vi "20220106_DO_Validation.vi"() -> ()   [LabVIEW 2021]
uses:
  <vilib>/Utility/file.llb/Read Delimited Spreadsheet (I64).vi
panel:
  out "Waveform Graph":waveform(i16)[](graph)
  out "Boolean array":bool[][](array[boolean])
  out "Waveform Chart":waveform(i64)(graph)
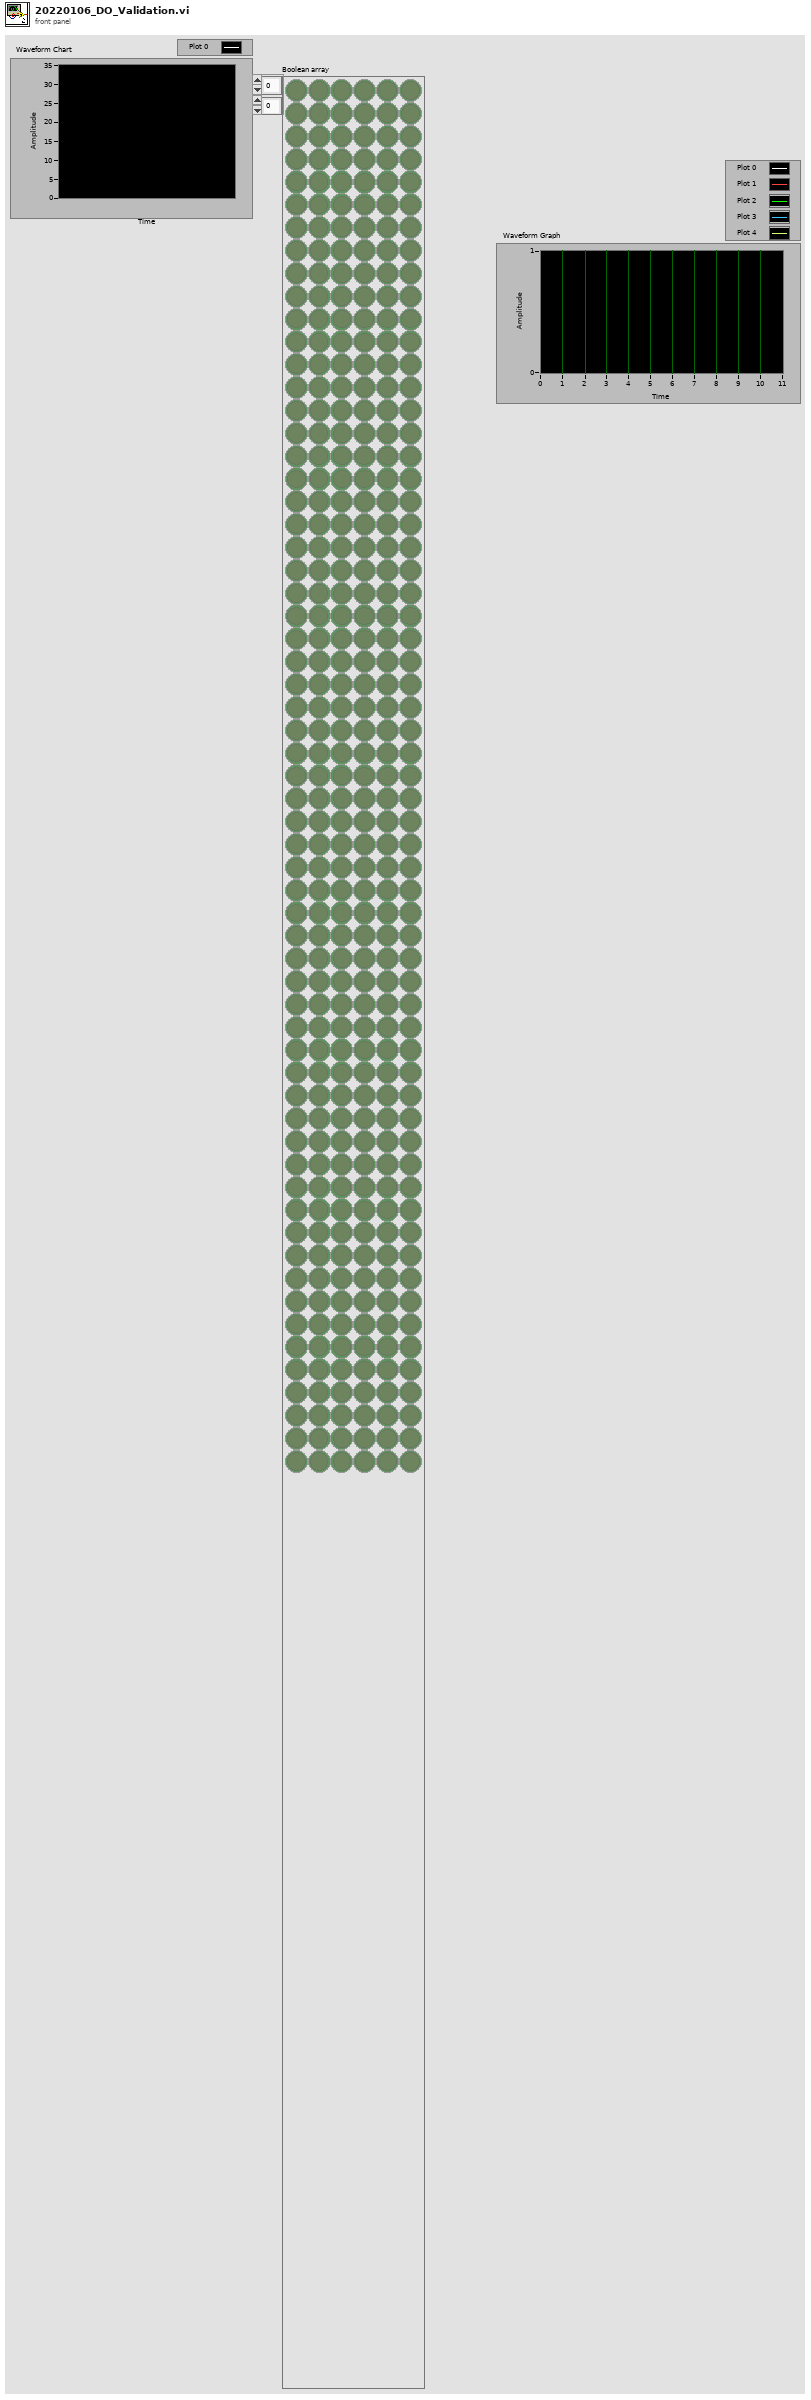
[diagram p1: front panel]
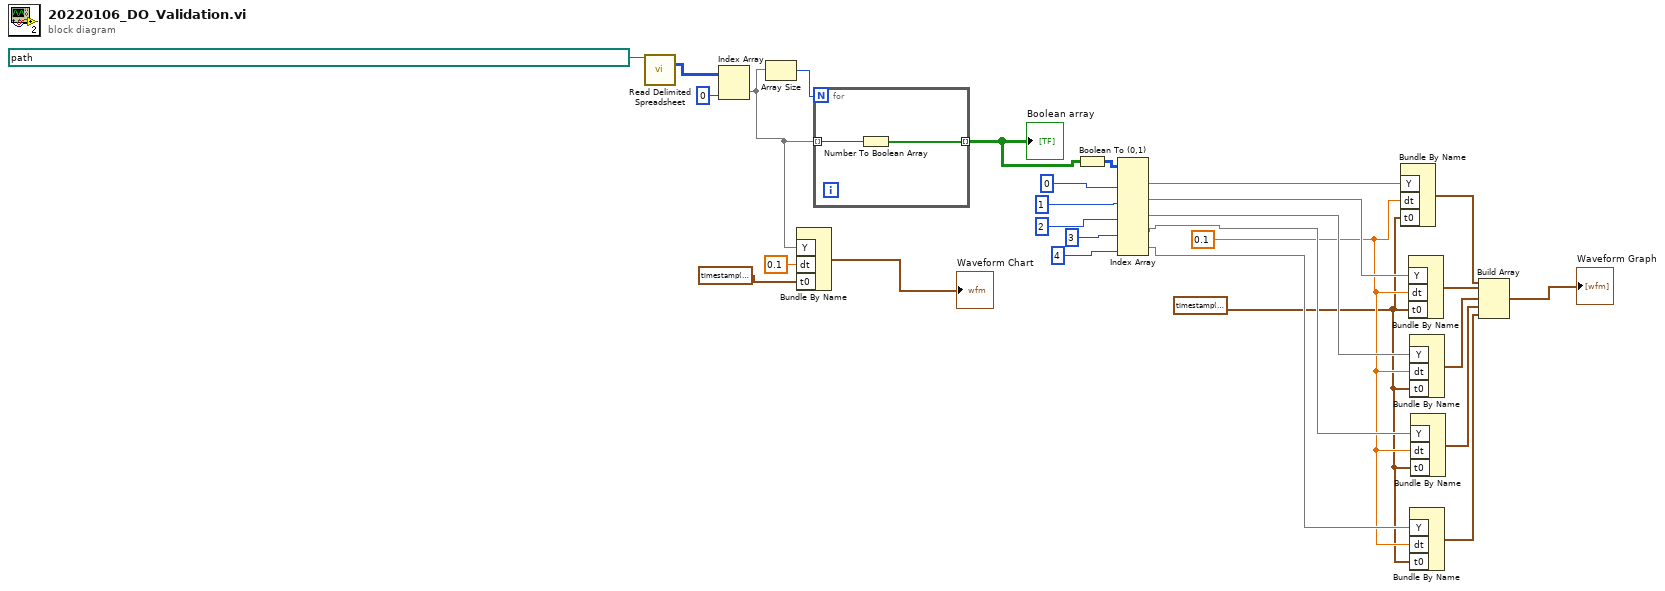
[diagram p0: block diagram]
diagram:
  w4 = timestamp(0 s since 1904-01-01) ("t0")
  w5 = 0.1 ("dt")
  n1 = call-poly <vilib>:"Read Delimited Spreadsheet.vi"("file path (dialog if empty)"=path "C:/Users/joe.kao/OneDrive - eCloudvalley Digital Technology/桌面/nPM1100_WaveformTable_Digital_LV.txt") -> ("all rows"=w27:i64[][])  [unwired: 9 in, 5 out]
  n2 = Index Array(array=w27, index (col)=0 ("disabled index (col)")) -> (element=w21:i64[])  [unwired: 1 in]
  n3 = Array Size(array=w21) -> (size(s)=w22:i32)
  n4 = Bundle By Name("Y"=w21, "dt"=0.1, "t0"=timestamp(0 s since 1904-01-01)) -> (→"Waveform Chart":waveform(i64))  [unwired: 1 in]
  n5 = for {
    N: w22 -> [_]
    tunnel: w21 -> [w30] mode=indexing
    tunnel: [w29] -> w15 mode=indexing
    n6 = Number To Boolean Array(number=w30) -> (Boolean array=w29:bool[])
  }
  "Boolean array" <- w15
  n7 = Boolean To (0,1)(Boolean=w15) -> (0, 1=w10:i16[][])
  n8 = Index Array(array=w10, index (col) #1=0 ("disabled index (col)"), index (col) #2=1 ("disabled index (row)"), index (col) #3=2 ("index (col)"), index (col) #4=3 ("index (col)"), index (col) #5=4 ("index (col)")) -> (element #1=w14:i16[], element #2=w13:i16[], element #3=w8:i16[], element #4=w7:i16[], element #5=w6:i16[])  [unwired: 5 in]
  n9 = Bundle By Name("Y"=w14, "dt"=w5, "t0"=w4) -> (w12:waveform(i16))  [unwired: 1 in]
  n10 = Bundle By Name("Y"=w13, "dt"=w5, "t0"=w4) -> (w9:waveform(i16))  [unwired: 1 in]
  n11 = Bundle By Name("Y"=w8, "dt"=w5, "t0"=w4) -> (w3:waveform(i16))  [unwired: 1 in]
  n12 = Bundle By Name("Y"=w6, "dt"=w5, "t0"=w4) -> (w1:waveform(i16))  [unwired: 1 in]
  n13 = Bundle By Name("Y"=w7, "dt"=w5, "t0"=w4) -> (w2:waveform(i16))  [unwired: 1 in]
  n14 = Build Array(w12, w9, w3, w2, w1) -> (→"Waveform Graph":waveform(i16)[])
